vi "Delete Math Expression.vi"(7 "Expression Name (Expression1)":string="Expression1", 8 "error in (no error)":errorcluster, 9 "Delete Operation (0: Delete One)":i32(ring) items=["Delete One", "Delete All"], 10 "Channel (1: Channel 1)":i32(ring)=1 items=["Channel 1"=1, "Channel 2"=2], 11 "VISA resource name":refnum<visa-resource-name>) -> (0 "error out":errorcluster, 3 "VISA resource name out":refnum<visa-resource-name>)   [LabVIEW 2012, in "Keysight B2980 Series.lvlib"]
doc: "Deletes one or all user-defined math expressions. This VI cannot delete predefined math expressions.\n\n<b>Note(s):</b>\nThis VI cannot delete predefined math expressions."
uses:
  Keysight B2980 Series.lvlib
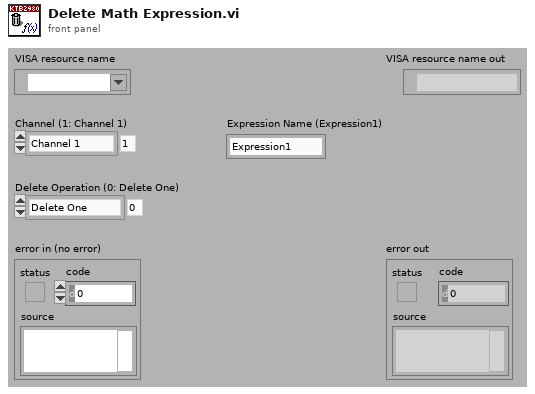
[diagram p1: front panel]
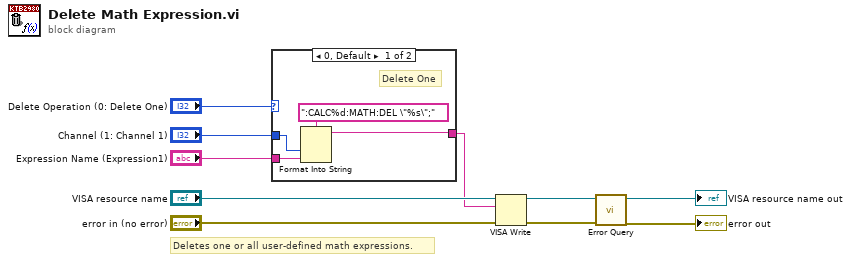
[diagram p0: block diagram]
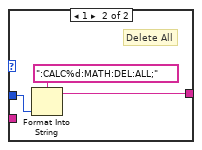
[diagram p2: hidden frame]
diagram:
  # "Deletes one or all user-defined math expressions."
  n1 = case shown="0, Default" "Delete Operation (0: Delete One)" {
    tunnel: "Channel (1: Channel 1)" -> [w13 w16]
    tunnel: "Expression Name (Expression1)" -> [w12 _]
    tunnel: [w11 w15] -> w1
    frame 0, Default {
      # "Delete One"
      n2 = Format Into String(format string=":CALC%d:MATH:DEL \"%s\";", w13, w12) -> (resulting string=w11:string)  [unwired: 2 in, 1 out]
    }
    frame 1 {
      # "Delete All"
      n3 = Format Into String(format string=":CALC%d:MATH:DEL:ALL;", w16) -> (resulting string=w15:string)  [unwired: 2 in, 1 out]
    }
  }
  n4 = VISA Write(VISA resource name="VISA resource name", write buffer=w1, error in (no error)="error in (no error)") -> (VISA resource name out=w7:refnum<visa-resource-name>, error out=w6:errorcluster)  [unwired: 1 out]
  n5 = call "Error Query.vi"("error in (no error)"=w6, "VISA resource name"=w7) -> ("error out"=→"error out":errorcluster, "VISA resource name out"=→"VISA resource name out":refnum<visa-resource-name>)  [unwired: 8 out]
